vi "get queue to manager.vi"(11 "connection in":refnum<class "connection maintainer.lvclass">) -> (3 "queue manager":refnum<class "identifying queue.lvclass">)   [LabVIEW 2015, in "connection maintainer.lvclass"]
uses:
  connection maintainer.lvclass
  communicator queue/identifying queue.lvclass
  connection maintainer.lvclass/connection maintainer.ctl
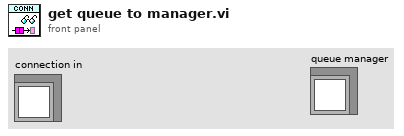
[diagram p1: front panel]
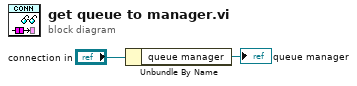
[diagram p0: block diagram]
diagram:
  n1 = Unbundle By Name("connection in") -> ("queue manager"=→"queue manager":refnum<class "identifying queue.lvclass">)
